vi "Initialize and Configure.vi"(8 "error in (no error)":errorcluster {"code" format="%.0x"}, 11 "VISA resource name":refnum<visa-resource-name>="GPIB::20") -> (0 "error out":errorcluster, 3 "VISA resource name out":refnum<visa-resource-name>)   [LabVIEW 2015]
panel:
  out "Catalog":string
  out "Trace List":string[][](array[string])
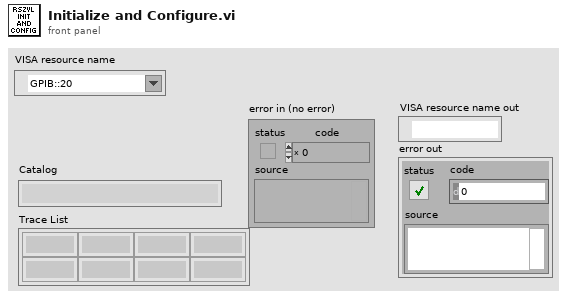
[diagram p1: front panel]
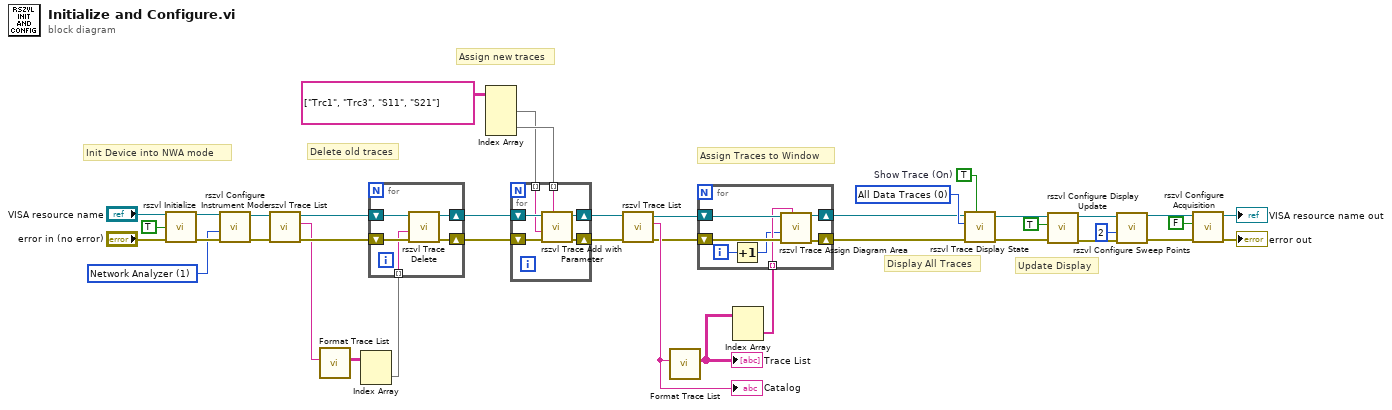
[diagram p0: block diagram]
diagram:
  w32 = TRUE  # Show Trace (On)
  w33 = 0 items=["All Data Traces", "All Memory Traces", "Single Trace"] ("Trace Type (All Data Traces)")
  w36 = 1 items=["Spectrum Analyzer", "Network Analyzer", "Noise Figure And Gain Measurements", "WCDMA Measurements", "WLAN OFDM Analysis", "WiMAX OFDM/OFDMA Analysis", "Analog Measurement Demodulator", "Bluetooth Measurements", "Cable TV Analyzer"] ("Instrument Mode (Network Analyzer)")
  # "Update Display"
  # "Assign Traces to Window"
  # "Assign new traces"
  # "Delete old traces"
  # "Display All Traces"
  # "Init Device into NWA mode"
  n1 = call <instrlib>:"rszvl Initialize.vi"("VISA resource name"="VISA resource name", "Reset (T: Reset)"=TRUE ("Reset (Reset)"), "error in (no error)"="error in (no error)") -> ("VISA resource name out"=w37:refnum<visa-resource-name>, "error out"=w38:errorcluster)  [unwired: 11 in]
  n2 = call <instrlib>:"rszvl Configure Instrument Mode.vi"("error in (no error)"=w38, "Instrument Mode (Network Analyzer)"=w36, "VISA resource name"=w37) -> ("error out"=w35:errorcluster, "VISA resource name out"=w34:refnum<visa-resource-name>)  [unwired: 7 in]
  n3 = call <instrlib>:"rszvl Trace List.vi"("error in (no error)"=w35, "VISA resource name"=w34) -> ("error out"=w22:errorcluster, "Catalog"=w19:string, "VISA resource name out"=w20:refnum<visa-resource-name>)  [unwired: 7 in]
  n4 = call "Format Trace List.vi"("Trace List Catalog"=w19) -> ("Trace List"=w12:string[][])  [unwired: 10 in]
  n5 = Index Array(array=w12) -> (element=w18:string[])  [unwired: 2 in]
  n6 = for {
    shift-right: [w44] -> w21
    shift-left: w22 -> [w45]
    shift-right: [w42] -> w17
    shift-left: w20 -> [w43]
    tunnel: w18 -> [w41] mode=indexing
    n7 = call <instrlib>:"rszvl Trace Delete.vi"("error in (no error)"=w45, "Trace Name (\"Trc1\")"=w41, "VISA resource name"=w43) -> ("error out"=w44:errorcluster, "VISA resource name out"=w42:refnum<visa-resource-name>)  [unwired: 7 in]
  }
  n8 = Index Array(array=string[][] [["Trc1", "Trc3"], ["S11", "S21"]] ("Trace List")) -> (element #1=w14:string[], element #2=w15:string[])  [unwired: 4 in]
  n9 = for {
    shift-right: [w50] -> w29
    shift-left: w21 -> [w51]
    shift-right: [w48] -> w28
    shift-left: w17 -> [w49]
    tunnel: w14 -> [w47] mode=indexing
    tunnel: w15 -> [w46] mode=indexing
    n10 = call <instrlib>:"rszvl Trace Add with Parameter.vi"("Parameter (\"S21\")"=w46, "error in (no error)"=w51, "Trace Name (\"Trc1\")"=w47, "VISA resource name"=w49) -> ("error out"=w50:errorcluster, "VISA resource name out"=w48:refnum<visa-resource-name>)  [unwired: 6 in]
  }
  n11 = call <instrlib>:"rszvl Trace List.vi"("error in (no error)"=w29, "VISA resource name"=w28) -> ("error out"=w26:errorcluster, "Catalog"=w27:string, "VISA resource name out"=w25:refnum<visa-resource-name>)  [unwired: 7 in]
  "Catalog" <- w27
  n12 = call "Format Trace List.vi"("Trace List Catalog"=w27) -> ("Trace List"=w24:string[][])  [unwired: 10 in]
  "Trace List" <- w24
  n13 = Index Array(array=w24) -> (element=w23:string[])  [unwired: 2 in]
  n14 = for {
    shift-right: [w57] -> w13
    shift-left: w26 -> [w58]
    shift-right: [w56] -> w30
    shift-left: w25 -> [w55]
    tunnel: w23 -> [w54] mode=indexing
    i -> [w53]
    n15 = Increment(x=w53) -> (x+1=w52:i32)
    n16 = call <instrlib>:"rszvl Trace Assign Diagram Area.vi"("Trace Name (\"Trc1\")"=w54, "error in (no error)"=w58, "Window (1)"=w52, "VISA resource name"=w55) -> ("error out"=w57:errorcluster, "VISA resource name out"=w56:refnum<visa-resource-name>)  [unwired: 6 in]
  }
  n17 = call <instrlib>:"rszvl Trace Display State.vi"("Show Trace (On)"=w32, "error in (no error)"=w13, "Trace Type (All Data Traces)"=w33, "VISA resource name"=w30) -> ("error out"=w10:errorcluster, "VISA resource name out"=w9:refnum<visa-resource-name>)  [unwired: 6 in]
  n18 = call <instrlib>:"rszvl Configure Display Update.vi"("error in (no error)"=w10, "Display Update (Off)"=TRUE, "VISA resource name"=w9) -> ("error out"=w8:errorcluster, "VISA resource name out"=w7:refnum<visa-resource-name>)  [unwired: 7 in]
  n19 = call <instrlib>:"rszvl Configure Sweep Points.vi"("error in (no error)"=w8, "Number Of Points (201)"=2, "VISA resource name"=w7) -> ("error out"=w1:errorcluster, "VISA resource name out"=w2:refnum<visa-resource-name>)  [unwired: 7 in]
  n20 = call <instrlib>:"rszvl Configure Acquisition.vi"("error in (no error)"=w1, "Sweep Mode Continuous (On)"=FALSE, "VISA resource name"=w2) -> ("error out"=→"error out":errorcluster, "VISA resource name out"=→"VISA resource name out":refnum<visa-resource-name>)  [unwired: 7 in]
